vi "Actor Core.vi"(8 "error in":errorcluster, 11 "Heater in":refnum<class "Heater.lvclass">) -> (0 "error out":errorcluster, 3 "Actor out":refnum<class "Actor.lvclass">)   [LabVIEW 2015, in "cRIO-Carbondioxide.lvlib" / "CO2-Actor.lvlib" / "Heater.lvclass"]
doc: "(<B>Filename</B>: Actor Framework.lvlib:Actor.lvclass:Actor Core.vi)\n\nReceives messages to the actor, reacts to them, and initiates any error handling that may shut the actor down.\n\nDescendant classes may override this VI to append parallel tasks for the actor to complete while it handles messages. Overrides use the Call Parent Method node."
uses:
  Heater.lvclass
  <vilib>/ActorFramework/Actor/Actor.lvclass
  <vilib>/ActorFramework/Actor/Actor.lvclass/Actor.ctl
  <vilib>/ActorFramework/Message Enqueuer/Message Enqueuer.lvclass/Message Enqueuer.ctl
  Heater.lvclass/Heater.ctl
  Heater Messages/Write Duty Cycle Msg/Write Duty Cycle Msg.lvclass/Write Duty Cycle Msg.ctl
  <vilib>/ActorFramework/Message Enqueuer/Enqueue.vi
  <vilib>/ActorFramework/Actor/Read Self Enqueuer.vi
  <vilib>/ActorFramework/Message Enqueuer/Init from Existing Queue.vi
  <vilib>/ActorFramework/Message Priority Queue/Priority Enqueue.vi
  CO2 Actor/CO2 Actor.lvclass
  <vilib>/ActorFramework/Message Enqueuer/Message Enqueuer.lvclass
  Heater Messages/Write Duty Cycle Msg/Write Duty Cycle Msg.lvclass
  <vilib>/ActorFramework/Stop Msg/Stop Msg.lvclass
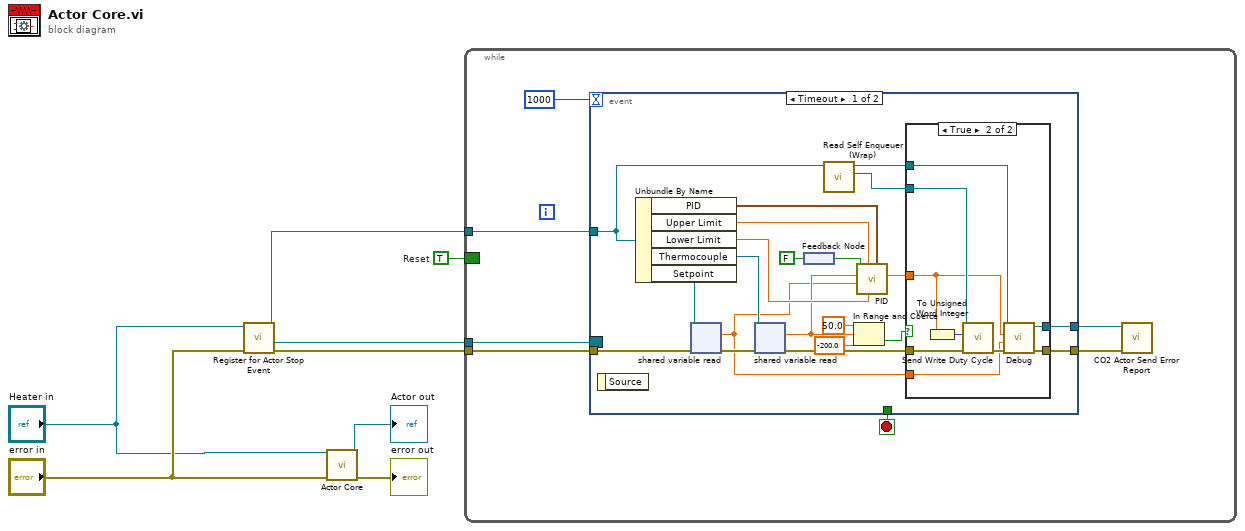
[diagram p0: block diagram]
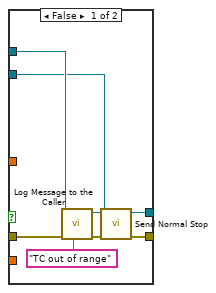
[diagram p2: hidden frame]
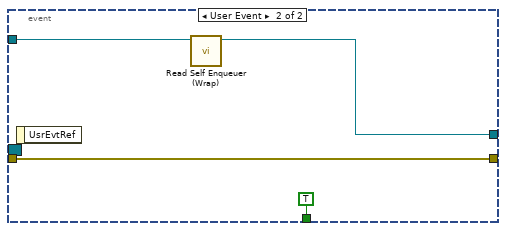
[diagram p3: hidden frame]
diagram:
  w7 = TRUE  # Reset
  n1 = call "Register for Actor Stop Event.vi"("error in (no error)"="error in", "CO2 Actor in"="Heater in") -> ("error out"=w5:errorcluster, "Event Registration Refnum"=w4:refnum<event-registration>, "CO2 Actor out"=w3:refnum<class "Heater.lvclass">)  [unwired: 7 in]
  n2 = call-parent "Actor Core.vi"("error in"="error in", "CO2 Actor in"="Heater in") -> ("error out"=→"error out":errorcluster, "Actor out"=→"Actor out":refnum<class "Actor.lvclass">)  [unwired: 8 in]
  n3 = while {
    tunnel: w4 -> [w14]
    tunnel: w5 -> [w12]
    tunnel: w3 -> [w11]
    border: w7 -> [_]
    stop <- w13 stop-if-true
    n4 = event shown="[0] Timeout" {
      selector: w14 -> [_ _]
      dyn-events: _ -> [_ _]
      timeout: 1000 -> [_ _]
      tunnel: [_ TRUE ("Actor Stop")] -> w13
      tunnel: w11 -> [w20 w55]
      tunnel: w12 -> [w23 w54]
      tunnel: [w34 w54] -> w10
      tunnel: [w16 w53] -> w9
      event Timeout {
        n5 = event-data() -> ()  [unwired: 1 in, 1 out]
        n6 = Unbundle By Name(w20) -> ("PID"=w36:cluster{"P":dbl, "I":dbl, "D":dbl}, "Upper Limit"=w32:dbl, "Lower Limit"=w30:dbl, "Thermocouple"=w25:refnum<k21>, "Setpoint"=w24:refnum<k21>)
        n7 = shared-variable-read(w24, w23) -> (w22:errorcluster, w17:dbl)  [unwired: 1 out]
        n8 = shared-variable-read(w25, w22) -> (w35:errorcluster, w26:dbl)  [unwired: 1 out]
        n9 = feedback-in #1(FALSE ("Reset")) -> ()
        n10 = feedback #1() -> (w21:bool)
        n11 = call "Read Self Enqueuer (Wrap).vi"("CO2 Actor in"=w20) -> ("Actor Framework:Message Enqueuer"=w18:refnum<class "Message Enqueuer.lvclass">, "CO2 Actor out"=w19:refnum<class "Heater.lvclass">)  [unwired: 9 in]
        n12 = In Range and Coerce(upper limit=50.0, x=w26, lower limit=-200.0) -> (In Range?=w27:bool)  [unwired: 1 out]
        n13 = call "PID.vi"("PID"=w36, "Lower Limit"=w30, "Upper Limit (0,01)"=w32, "Setpoint (0,002)"=w17, "Process"=w26, "Reset"=w21) -> ("Output"=w31:dbl)  [unwired: 4 in, 1 out]
        n14 = case shown="True" w27 {
          tunnel: w35 -> [w42 w52]
          tunnel: [w43 w48] -> w34
          tunnel: w31 -> [_ w46]
          tunnel: w18 -> [w38 w50]
          tunnel: w19 -> [w39 w47]
          tunnel: [w37 w44] -> w16
          tunnel: w17 -> [_ w45]
          frame False {
            n15 = call-dynamic "Log Message to the Caller.vi"("String (\"\" = no message to send)"="TC out of range", "error in (no error)"=w42, "CO2 Actor in"=w39) -> ("error out"=w40:errorcluster, "CO2 Actor out"=w37:refnum<class "Heater.lvclass">)  [unwired: 7 in]
            n16 = call <vilib>:"Send Normal Stop.vi"("error in (no error)"=w40, "Message Enqueuer"=w38) -> ("error out"=w43:errorcluster)  [unwired: 9 in]
          }
          frame True {
            n17 = To Unsigned Word Integer(number=w46) -> (unsigned 16bit integer=w51:u16)
            n18 = call "Send Write Duty Cycle.vi"("error in (no error)"=w52, "Duty Cycle (0‰)"=w51, "Message Enqueuer"=w50) -> ("error out"=w49:errorcluster)  [unwired: 7 in, 1 out]
            n19 = call "Debug.vi"("error in (no error)"=w49, "Numeric 1"=w45, "Numeric 0"=w46, "Heater in"=w47) -> ("error out"=w48:errorcluster, "Heater out"=w44:refnum<class "Heater.lvclass">)  [unwired: 6 in]
          }
        }
      }
      event User Event {
        n20 = event-data() -> ()  [unwired: 1 in, 1 out]
        n21 = call "Read Self Enqueuer (Wrap).vi"("CO2 Actor in"=w55) -> ("CO2 Actor out"=w53:refnum<class "Heater.lvclass">)  [unwired: 9 in, 1 out]
      }
    }
    n22 = call-dynamic "CO2 Actor Send Error Report.vi"("Error From Sender"=w10, "CO2 Actor in"=w9) -> ()  [unwired: 9 in, 1 out]
  }
